vi "Write waveform.vi"(4 "Channel":string="wave", 6 "Name note":string="Блок формирования кадра", 8 "error in (no error)":errorcluster, 10 "Waveform":waveform(dbl)) -> (0 "error out":errorcluster)   [LabVIEW 2019]
uses:
  <vilib>/addons/_NIFileIO/SV TDMS Write Waveform (1 Ch).vi
  <vilib>/Utility/config.llb/Write Key (Double).vi
  <vilib>/Utility/config.llb/NI_LVConfig.lvlib
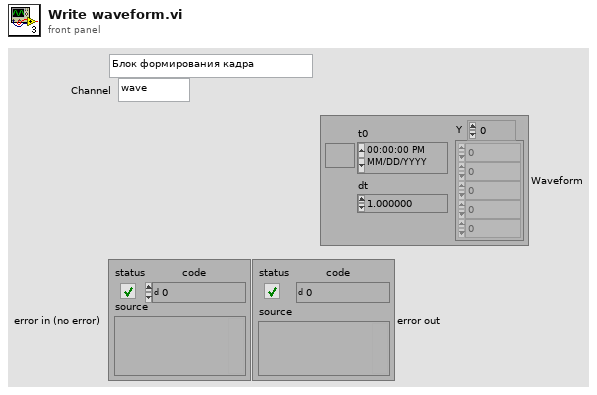
[diagram p1: front panel]
types:
  T1 = enum16{"fractional", "engineering", "exponential"}
  T2 = enum16{"open", "open or create", "create or replace", "create", "open (read-only)"}
  T3 = typedef "NI_LVConfig.lvlib/Config Data RefNum.ctl" = refnum<k1>
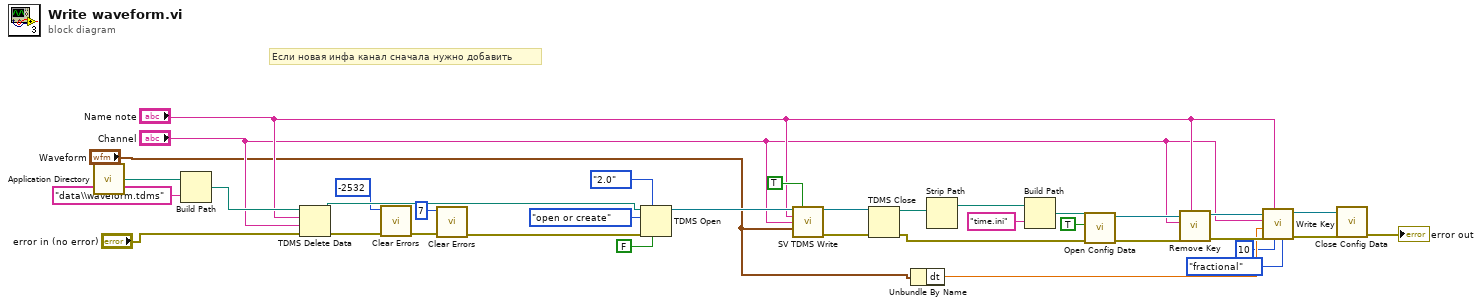
[diagram p0: block diagram]
diagram:
  # "Если новая инфа канал сначала нужно добавить"
  n1 = call <vilib>:"Application Directory.vi"() -> ("Application Directory"=w35:path)
  n2 = Build Path(base path=w35, name or relative path="data\\waveform.tdms") -> (appended path=w32:path)
  n3 = TDMS Delete Data(8:"error in (no error)", 9:"Channel", 10:"Name note", 11:w32) -> (0:w30:errorcluster, 3:w31:path)  [unwired: 3 in]
  n4 = call <vilib>:"Clear Errors.vi"("error in (no error)"=w30, "specific error code to clear (0: all)"=-2532) -> ("error out"=w28:errorcluster)  [unwired: 4 in, 1 out]
  n5 = call <vilib>:"Clear Errors.vi"("error in (no error)"=w28, "specific error code to clear (0: all)"=7) -> ("error out"=w27:errorcluster)  [unwired: 4 in, 1 out]
  n6 = TDMS Open(6:FALSE ("disable buffering? (T)"), 7:enum16{"1.0", "2.0"}."2.0" ("file format version (2.0)"), 8:w27, 10:T2."open or create" ("operation (0:open)"), 11:w31) -> (3:w23:refnum<k34>)  [unwired: 2 in, 1 out]
  n7 = call-poly <vilib>:"SV TDMS Write.vi"("tdms file"=w23, "write channel properties (T)"=TRUE, "group name in"="Name note", "channel name in"="Channel", "scaled signal [EU]"="Waveform") -> ("tdms file out"=w21:refnum<k34>, "error out"=w20:errorcluster)  [unwired: 7 in, 2 out]
  n8 = TDMS Close(8:w20, 11:w21) -> (0:w14:errorcluster, 3:w19:path)
  n9 = Unbundle By Name("Waveform") -> ("dt"=w6:dbl)
  n10 = Strip Path(path=w19) -> (stripped path=w18:path)  [unwired: 1 out]
  n11 = Build Path(base path=w18, name or relative path="time.ini") -> (appended path=w16:path)
  n12 = call <vilib>:"Open Config Data.vi"("error in (no error)"=w14, "create file if necessary (T)"=TRUE, "configuration file path"=w16) -> ("error out"=w13:errorcluster, "refnum"=w12:T3)  [unwired: 6 in, 1 out]
  n13 = call <vilib>:"Remove Key.vi"("section"="Name note", "error in (no error)"=w13, "key"="Channel", "refnum"=w12) -> ("error out"=w10:errorcluster, "refnum out"=w11:T3)  [unwired: 5 in, 1 out]
  n14 = call-poly <vilib>:"Write Key.vi"("format (fractional)"=T1."fractional", "precision (6)"=i16 10, "section"="Name note", "error in (no error)"=w10, "value"=w6, "key"="Channel", "refnum"=w11) -> ("error out"=w3:errorcluster, "refnum out"=w2:T3)  [unwired: 2 in, 1 out]
  n15 = call <vilib>:"Close Config Data.vi"("error in (no error)"=w3, "refnum"=w2) -> ("error out"=→"error out":errorcluster)  [unwired: 8 in, 1 out]
